vi "InfraredEmitter.vi"() -> ()   [LabVIEW 2024]
uses:
  Driver/Public/Digital Direction.ctl
  Driver/CTIPicoVISA.lvlib
panel:
  out "Boolean":bool
  out "Identity":T1
  in  "GroveConnector":enum16{"D16", "D18", "D20"}(ring)
  in  "stop":bool
  in  "VISA resource name in":refnum<visa-resource-name>
  out "error out":errorcluster
  # "https://wiki.seeedstudio.com/Grove-Infrared_Emitter/"
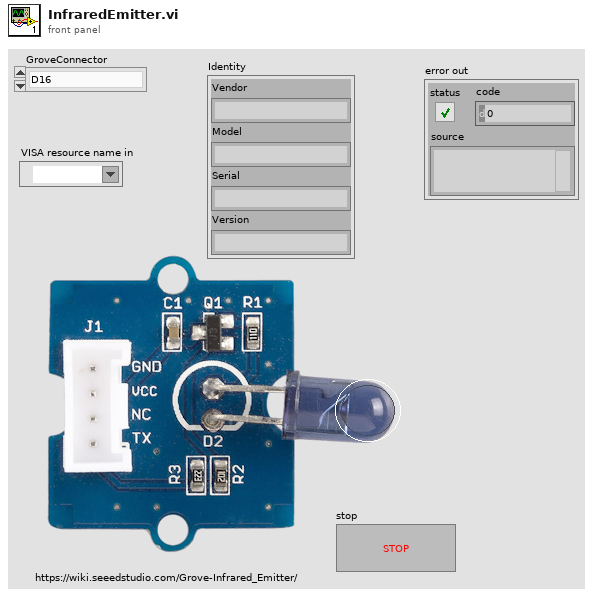
[diagram p1: front panel]
types:
  T1 = cluster{"Vendor":string, "Model":string, "Serial":string, "Version":string}
  T2 = typedef "CTIPicoVISA.lvlib/Digital Direction.ctl" = enum16{"In", "Out"}
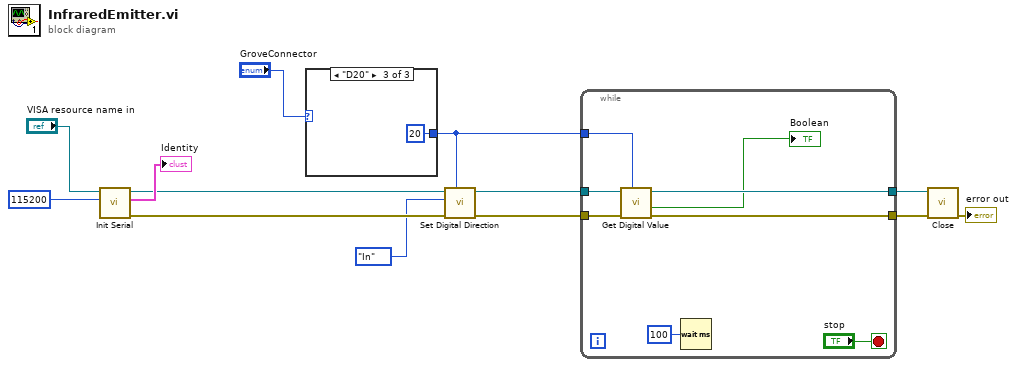
[diagram p0: block diagram]
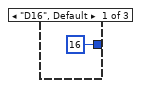
[diagram p2: hidden frame]
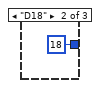
[diagram p3: hidden frame]
diagram:
  n1 = call "Init Serial.vi"("Baud (115200)"=u32 115200, "VISA resource name in"="VISA resource name in") -> ("error out"=w7:errorcluster, "Identity"=→"Identity":T1, "VISA resource name Out"=w9:refnum<visa-resource-name>)  [unwired: 7 in]
  n2 = case shown="\"D20\"" "GroveConnector" {
    tunnel: [16 ("GPIO") 18 ("GPIO") 20 ("GPIO")] -> w8
    frame "D16", Default {
    }
    frame "D18" {
    }
    frame "D20" {
    }
  }
  n3 = call "Set Digital Direction.vi"("GPIO"=w8, "error in (no error)"=w7, "Direction"=Digital_Direction."In", "VISA resource name in"=w9) -> ("error out"=w2:errorcluster, "VISA resource name"=w1:refnum<visa-resource-name>)  [unwired: 6 in]
  n4 = while {
    tunnel: w2 -> [w20]
    tunnel: w1 -> [w21]
    tunnel: [w19] -> w5
    tunnel: [w18] -> w4
    tunnel: w8 -> [w22]
    stop <- "stop" stop-if-true
    n5 = call "Get Digital Value.vi"("GPIO"=w22, "error in (no error)"=w20, "VISA resource name in"=w21) -> ("error out"=w18:errorcluster, "Value"=→"Boolean":bool, "VISA resource name"=w19:refnum<visa-resource-name>)  [unwired: 6 in]
    n6 = Wait (ms)(milliseconds to wait=u32 100) -> ()  [unwired: 1 out]
  }
  n7 = call "Close.vi"("error in (no error)"=w4, "VISA resource name in"=w5) -> ("error out"=→"error out":errorcluster)  [unwired: 9 in]
